vi "Parse HW Tree.vi"(5 "Initial Index":i32, 6 "Depth":i32, 7 "Parent Index (None)":i32=-1, 8 "error in (no error)":errorcluster, 10 "JSON":string) -> (0 "error out":errorcluster, 2 "Nodes":T1[](array[typedef]))   [LabVIEW 2022 SP3, in "open-hw-mon-lv.lvlib" / "OpenHW.lvclass"]
uses:
  OpenHW.lvclass
  HW Node.ctl
  OpenHW.lvclass/OpenHW.ctl
  <vilib>/IlluminatedG/lv-web-crypto/lv-json/JSON/JSON.lvlib
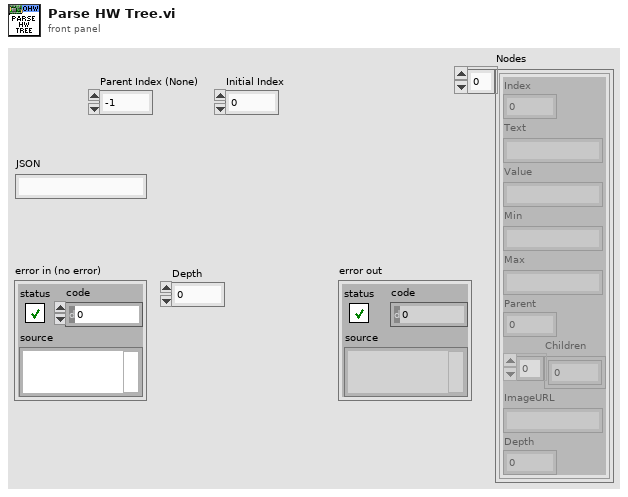
[diagram p1: front panel]
types:
  T1 = typedef "open-hw-mon-lv.lvlib/OpenHW.lvclass/HW Node.ctl" = cluster{"Index":i32, "Text":string, "Value":string, "Min":string, "Max":string, "Parent":i32, "Children":i32[], "ImageURL":string, "Depth":i32}
  T2 = typedef "JSON.lvlib/JSON Item Type.ctl" = enum16{"unknown", "null", "Array", "Object", "String", "Number", "Boolean"}
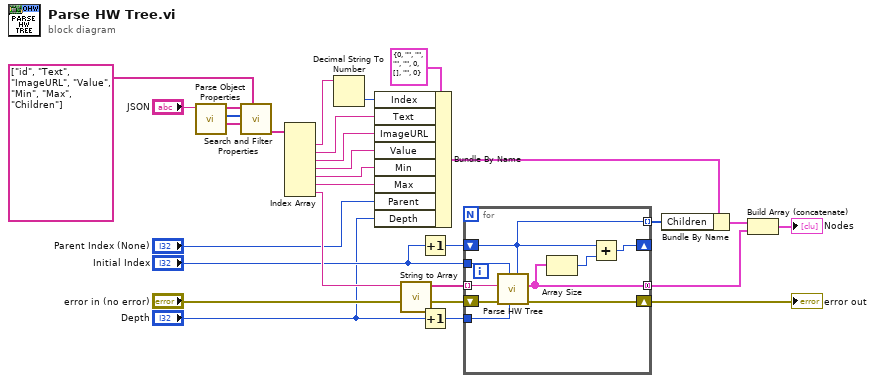
[diagram p0: block diagram]
diagram:
  n1 = call <vilib>:"Parse Object Properties.vi"("JSON String"="JSON") -> ("Values"=w25:string[], "Item Types"=w26:T2[], "Keys"=w27:string[])  [unwired: 7 in, 1 out]
  n2 = call <vilib>:"Search and Filter Properties.vi"("Search Keys"=string[] ["id", "Text", "ImageURL", "Value", "Min", "Max", "Children"], "Values In"=w25, "Types In"=w26, "Keys In"=w27) -> ("Filtered Values"=w24:string[])  [unwired: 2 in, 5 out]
  n3 = Index Array(array=w24) -> (element #1=w23:string, element #2=w20:string, element #3=w19:string, element #4=w18:string, element #5=w17:string, element #6=w16:string, element #7=w15:string)  [unwired: 7 in]
  n4 = Decimal String To Number(string=w23) -> (number=w21:i32)  [unwired: 2 in, 1 out]
  n5 = Bundle By Name(cluster=T1 {"Index"=0, "Text"="", "Value"="", "Min"="", "Max"="", "Parent"=0, "Children"=[], "ImageURL"="", "Depth"=0} ("HW Node"), "Index"=w21, "Text"=w20, "ImageURL"=w19, "Value"=w18, "Min"=w17, "Max"=w16, "Parent"="Parent Index (None)", "Depth"="Depth") -> (w9:T1)
  n6 = call <vilib>:"String to Array.vi"("Array String In"=w15) -> ("JSON Strings"=w14:string[])  [unwired: 10 in]
  n7 = Increment(x="Initial Index") -> (x+1=w4:i32)
  n8 = Increment(x="Depth") -> (x+1=w2:i32)
  n9 = for {
    tunnel: w14 -> [w37] mode=indexing
    tunnel: "Initial Index" -> [w36]
    shift-right: [w33] -> _
    shift-left: w4 -> [w30]
    tunnel: [w35] -> w8 mode=concatenating
    shift-right: [w31] -> w10
    shift-left: "error in (no error)" -> [w32]
    tunnel: [w30] -> w5 mode=indexing
    tunnel: w2 -> [w29]
    n10 = call "Parse HW Tree.vi"("Initial Index"=w30, "Depth"=w29, "Parent Index (None)"=w36, "error in (no error)"=w32, "JSON"=w37) -> ("error out"=w31:errorcluster, "Nodes"=w35:T1[])  [unwired: 5 in]
    n11 = Array Size(array=w35) -> (size(s)=w34:i32)
    n12 = Add(x=w30, y=w34) -> (x+y=w33:i32)
  }
  "error out" <- w10
  n13 = Bundle By Name(cluster=w9, "Children"=w5) -> (w6:T1)
  n14 = Build Array (concatenate)(w6, w8) -> (→"Nodes":T1[])
